vi "计算直线的斜率与截距.vi"(8 "Error In":errorcluster caption="错误输入", 10 "点B":T2, 11 "点A":T2) -> (0 "Error Out":errorcluster caption="错误输出", 3 "斜率与截距":T1)   [LabVIEW 2012, in "几何工具.lvlib"]
uses:
  <vilib>/Utility/miscctls.llb/LVPointDoubleTypeDef.ctl
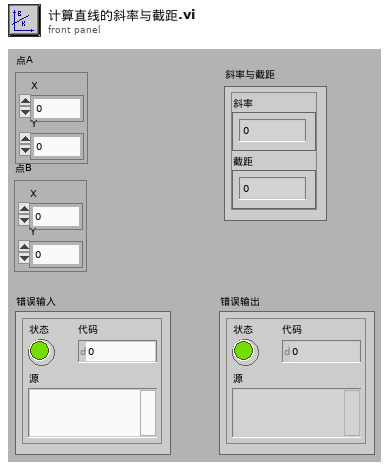
[diagram p1: front panel]
types:
  T1 = typedef "几何工具.lvlib/斜率与截距.ctl" = cluster{"斜率":dbl, "截距":dbl}
  T2 = typedef "LVPointDoubleTypeDef.ctl" = cluster{"X":dbl, "Y":dbl}
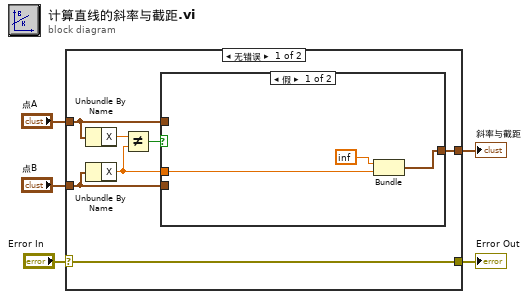
[diagram p0: block diagram]
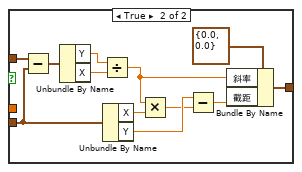
[diagram p2: hidden frame]
diagram:
  n1 = case shown="无错误" "Error In" {
    selector: "Error In" -> [w11 w28]
    tunnel: [w11 w28] -> w4
    tunnel: "点A" -> [w10 _]
    tunnel: "点B" -> [w9 _]
    tunnel: [w12 _] -> w1
    frame No Error {
      n2 = Unbundle By Name(w10) -> ("X"=w8:dbl)
      n3 = Unbundle By Name(w9) -> ("X"=w6:dbl)
      n4 = Not Equal?(x=w8, y=w6) -> (x != y?=w7:bool)
      n5 = case shown="假" w7 {
        tunnel: w10 -> [_ w18]
        tunnel: w9 -> [_ w17]
        tunnel: [w15 w16] -> w12
        tunnel: w6 -> [w13 _]
        frame False {
          n6 = Bundle("X"=inf, "X"=w13) -> (w15:cluster{"X":dbl, "X":dbl})  [unwired: 1 in]
        }
        frame True {
          n7 = Subtract(x=w18, y=w17) -> (x-y=w27:T2)
          n8 = Unbundle By Name(w27) -> ("Y"=w26:dbl, "X"=w25:dbl)
          n9 = Divide(x=w26, y=w25) -> (x/y=w20:dbl)
          n10 = Unbundle By Name(w17) -> ("X"=w24:dbl, "Y"=w23:dbl)
          n11 = Multiply(x=w20, y=w24) -> (x*y=w22:dbl)
          n12 = Subtract(x=w23, y=w22) -> (x-y=w19:dbl)
          n13 = Bundle By Name(cluster=T1 {"斜率"=0.0, "截距"=0.0} ("输出簇"), "斜率"=w20, "截距"=w19) -> (w16:T1)
        }
      }
    }
    frame Error {
    }
  }
  "Error Out" <- w4
  "斜率与截距" <- w1
